vi "FPGA IO.vi"() -> ()   [LabVIEW 2012]
doc: "Accepts inputs from a host based VI for controlling analog and digital outputs on a R-series board containing an FPGA. This VI will produce 4 different signal types dependent on the user input and the channel of interest. When the <B>WaveType</B> is set to laser, the first three channels will produce either a sine or square wave at the frequency <B>f0</B> while the last two produce only square waves. When the wavetype is set to speaker or none, all channels produce the same signal (although for the speaker, signals with a gain of <B>Amp</B> applied)."
uses:
  <vilib>/Platform/TimedLoop/XDataNode/XDataNode.xnode
  <vilib>/Platform/TimedLoop/XDataNode/nitl_modes.ctl
  <vilib>/Platform/TimedLoop/XDataNode/XDNodeRunTimeDep.lvlib
  <vilib>/Platform/TimedLoop/XDataNode/wakeup.ctl
  <vilib>/Platform/TimedLoop/XDataNode/timing_clust.ctl
  <vilib>/eio/EIONode/EIONode.xnode
  <vilib>/rvi/FXPMathLib/FxpMul/XNode/nifxpmath_Multiplier.xnode
  <vilib>/rvi/FXPMathLib/FxpAdd/XNode/nifxpmath_Add.xnode
  <vilib>/rvi/eio/common/nirviEmuTemplateMethod_errors.vi
  <vilib>/rvi/FXPMathLib/sim/FxpSim.dll
  Controls/FxdPt Props.ctl
  Controls/FPGA Signal.ctl
  Reusable/PAS/Main/Controls/Laser Modulation.ctl
panel:
  in  "LaserEn":T1
  in  "Laser Switch":bool
  out "OtherOut":T2
  in  "Cell 5":T3
  in  "Cell 4":T3
  in  "Cell 3":T3
  in  "Cell 2":T3
  in  "Cell 1":T3
  in  "wType":T5
  out "Stopped":bool
  out "SquareOut":T2
  in  "stop":bool
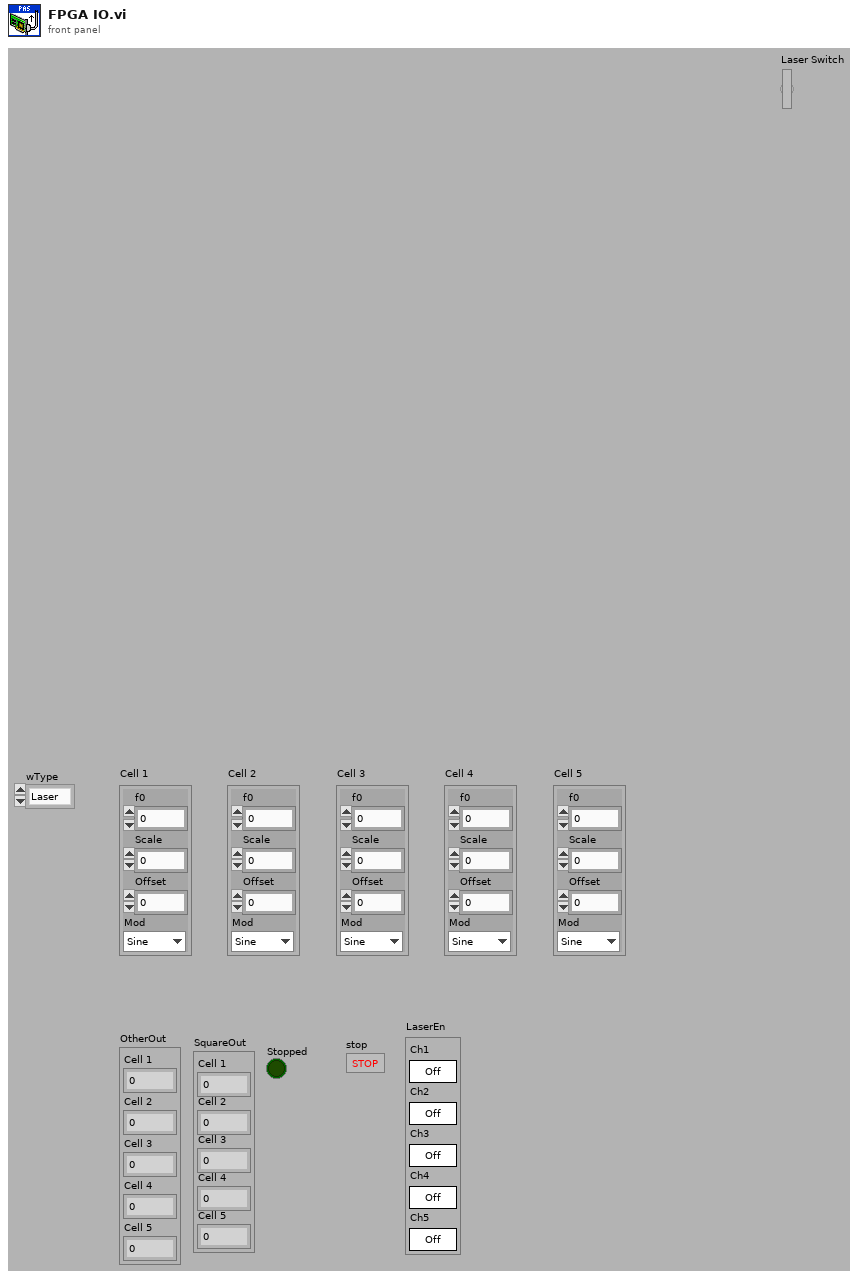
[diagram p1: front panel]
types:
  T1 = cluster{"Ch1":bool, "Ch2":bool, "Ch3":bool, "Ch4":bool, "Ch5":bool}
  T2 = cluster{"Cell 1":i16, "Cell 2":i16, "Cell 3":i16, "Cell 4":i16, "Cell 5":i16}
  T3 = typedef "FxdPt Props.ctl" = cluster{"f0":fxp<+,32,0>, "Scale":fxp<+,14,1>, "Offset":i16, "Mod":T4}
  T4 = typedef "Laser Modulation.ctl" = enum8{"Sine", "Square"}
  T5 = typedef "FPGA Signal.ctl" = enum16{"Laser", "None", "Speaker"}
  T6 = typedef "XDNodeRunTimeDep.lvlib/timing_clust.ctl" = cluster{"Expected End [f-1]":u64, "Actual End [f-1]":u64, "Finished Late? [f-1]":bool, "Expected End [i-1]":u64, "Actual End [i-1]":u64, "Finished Late? [i-1]":bool, "Expected Start [i]":u64, "Actual Start [i]":u64, "Expected Start [f]":u64, "Actual Start [f]":u64, "Source Name":string, "Structure Name":string, "Period":i64, "Deadline":i64, "Offset":i64, "Start":i64, "Priority":i32, "Timeout":i32, "Mode":T7, "Wakeup Reason":T8, "Error":errorcluster, "Source Type":string, "Secondary Source Type":string, "Global End Time":u64, "Global Start Time":u64, "Frame Duration":u64, "Iteration Duration":u64, "Assigned CPU":i32, "I/O Scan Engine Mode":u32}
  T7 = typedef "XDNodeRunTimeDep.lvlib/nitl_modes.ctl" = enum32{"No Change", "Process missed periods, maintain original phase", "Discard missed periods, maintain original phase", "Process missed periods, ignore original phase", "Discard missed periods, ignore original phase"}
  T8 = typedef "XDNodeRunTimeDep.lvlib/wakeup.ctl" = enum32{"Normal", "Aborted", "Asynchronous wakeup", "Timing source error", "Timed loop error", "Timeout"}
  T9 = cluster{"square wave out":i16, "square wave out":i16, "square wave out":i16, "square wave out":i16, "square wave out":i16}
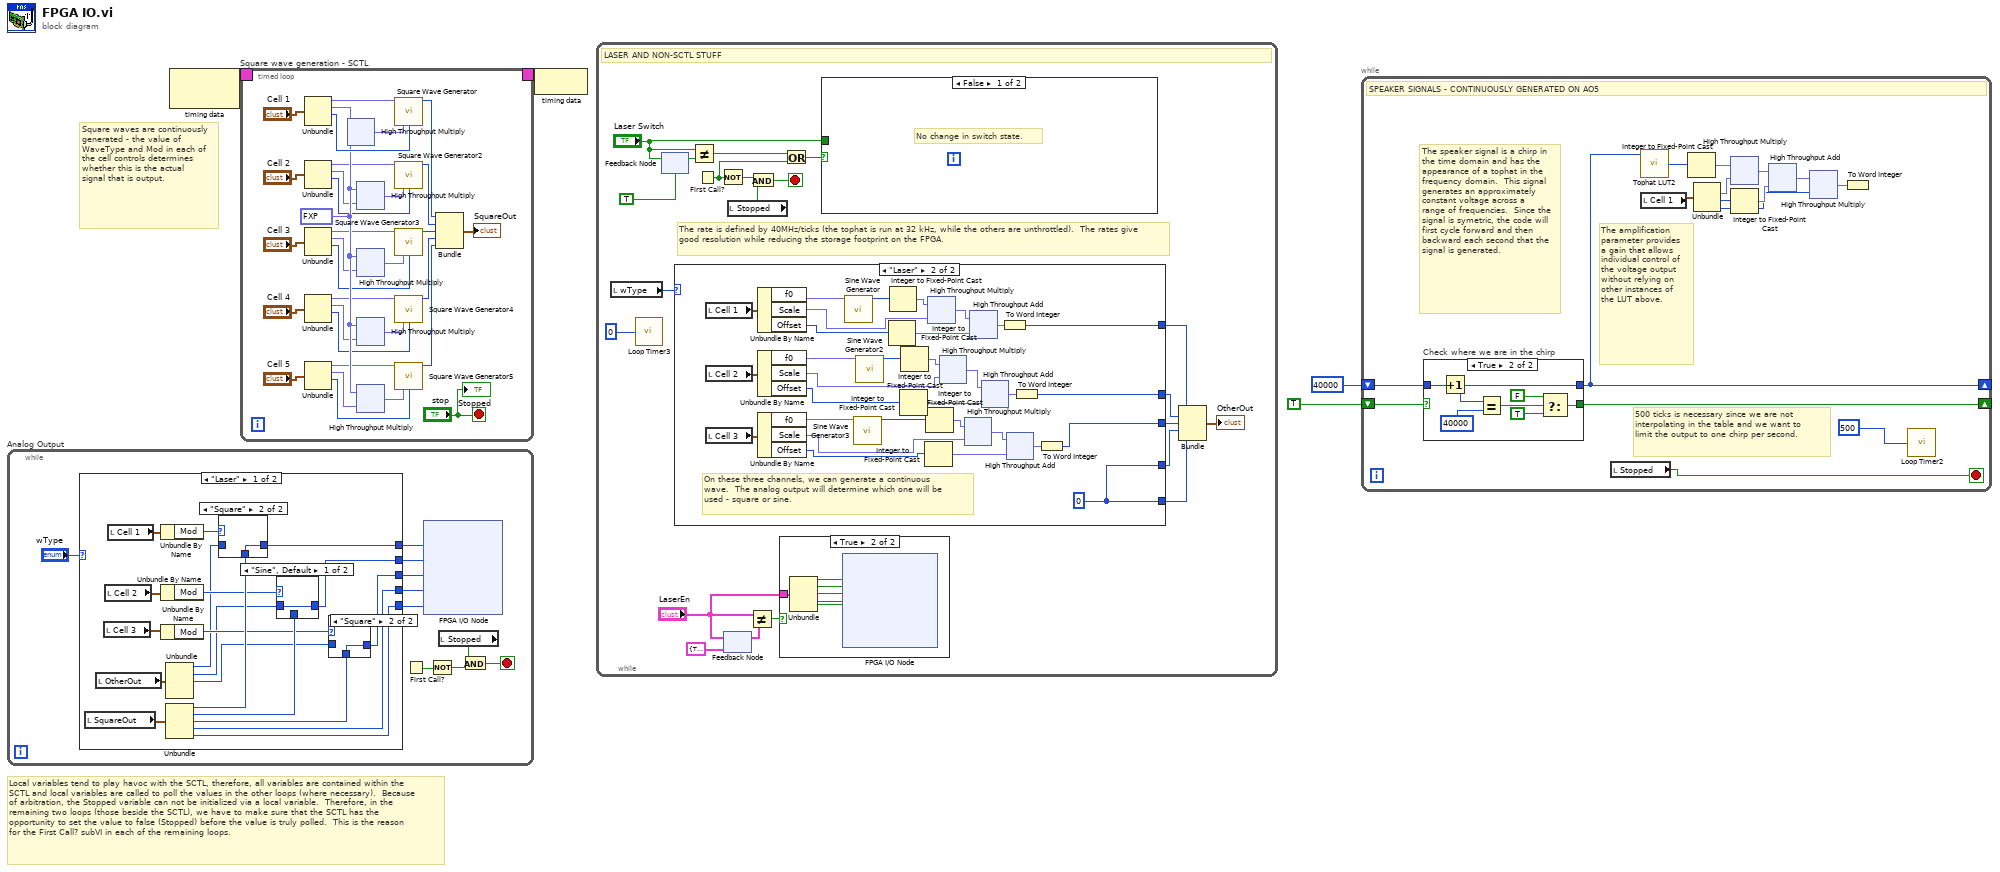
[diagram p0: block diagram]
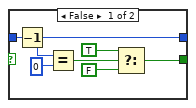
[diagram p2: hidden frame]
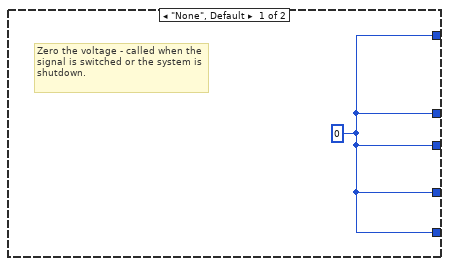
[diagram p4: hidden frame]
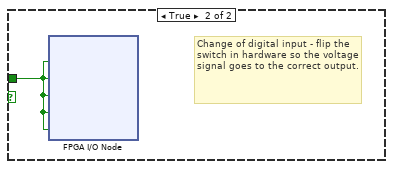
[diagram p5: hidden frame]
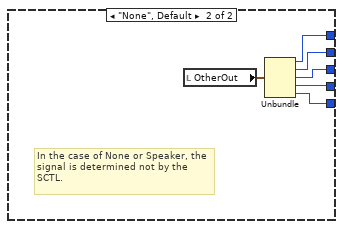
[diagram p9: hidden frame]
diagram:
  # "Square waves are continuously generated - the value of WaveType and Mod in each of the cell controls determines whether this is the actual signal that is output."
  # "Local variables tend to play havoc with the SCTL, therefore, all variables are contained within the SCTL and local variables are called to poll the values in the other loops (where necessary).  Because of arbitration, the Stopped variable can not be initialized via a local variable.  Therefore, in the remaining two loops (those beside the SCTL), we have to make sure that the SCTL has the opportunity to set the value to false (Stopped) before the value is truly polled.  This is the reason for the First Call? subVI in each of the remaining loops."
  n1 = while "Analog Output" {
    stop <- w5 stop-if-true
    n2 = case shown="\"Laser\"" "wType" {
      tunnel: [w26 w44] -> w14
      tunnel: [w16 w43] -> w13
      tunnel: [w15 w42] -> w12
      tunnel: [w31 w41] -> w11
      tunnel: [w32 w40] -> w10
      frame "Laser" {
        n3 = local read "SquareOut"() -> (w33:T2)
        n4 = local read "OtherOut"() -> (w30:T2)
        n5 = local read "Cell 3"() -> (w22:T3)
        n6 = local read "Cell 2"() -> (w24:T3)
        n7 = local read "Cell 1"() -> (w29:T3)
        n8 = Unbundle By Name(w29) -> ("Mod"=w28:T4)
        n9 = Unbundle By Name(w24) -> ("Mod"=w23:T4)
        n10 = Unbundle By Name(w22) -> ("Mod"=w21:T4)
        n11 = Unbundle(w30) -> ("Cell 1"=w17:i16, "Cell 2"=w18:i16, "Cell 3"=w19:i16)  [unwired: 2 out]
        n12 = Unbundle(w33) -> ("Cell 1"=w27:i16, "Cell 2"=w25:i16, "Cell 3"=w20:i16, "Cell 4"=w31:i16, "Cell 5"=w32:i16)
        n13 = case shown="\"Square\"" w28 {
          tunnel: w27 -> [_ w39]
          tunnel: [w38 w39] -> w26
          tunnel: w17 -> [w38 _]
          frame "Sine", Default {
          }
          frame "Square" {
          }
        }
        n14 = case shown="\"Sine\", Default" w23 {
          tunnel: w25 -> [_ w37]
          tunnel: [w36 w37] -> w16
          tunnel: w18 -> [w36 _]
          frame "Sine", Default {
          }
          frame "Square" {
          }
        }
        n15 = case shown="\"Square\"" w21 {
          tunnel: w20 -> [_ w35]
          tunnel: [w34 w35] -> w15
          tunnel: w19 -> [w34 _]
          frame "Sine", Default {
          }
          frame "Square" {
          }
        }
      }
      frame "None", Default {
        # "In the case of None or Speaker, the signal is determined not by the SCTL."
        n16 = local read "OtherOut"() -> (w45:T2)
        n17 = Unbundle(w45) -> ("Cell 1"=w44:i16, "Cell 2"=w43:i16, "Cell 3"=w42:i16, "Cell 4"=w41:i16, "Cell 5"=w40:i16)
      }
    }
    n18 = First Call?() -> (First Call?: T/F=w8:bool)
    n19 = xnode "FPGA I/O Node"("Ch 1 AO"=w14, "Ch 2 AO"=w13, "Ch 3 AO"=w12, "Ch 4 AO"=w11, "Ch 5 AO"=w10) -> ()  [unwired: 5 in, 5 out]
    n20 = Not(x=w8) -> (.not. x?=w6:bool)
    n21 = local read "Stopped"() -> (w7:bool)
    n22 = And(x=w7, y=w6) -> (x .and. y?=w5:bool)
  }
  n23 = node-c288() -> (w4:T6)  [unwired: 1 in]
  n24 = timed-loop "Square wave generation - SCTL" {
    timing: w4 -> [_]
    timing-out: [_] -> w3
    stop <- "stop" stop-if-true
    w66 = fxp<+,15,15> 32767.0 ("n")
    n25 = Unbundle("Cell 1") -> ("f0"=w69:fxp<+,32,0>, "Scale"=w68:fxp<+,14,1>, "Offset"=w67:i16)  [unwired: 1 out]
    n26 = Unbundle("Cell 2") -> ("f0"=w57:fxp<+,32,0>, "Scale"=w56:fxp<+,14,1>, "Offset"=w58:i16)  [unwired: 1 out]
    n27 = Unbundle("Cell 3") -> ("f0"=w54:fxp<+,32,0>, "Scale"=w55:fxp<+,14,1>, "Offset"=w59:i16)  [unwired: 1 out]
    n28 = Unbundle("Cell 4") -> ("f0"=w53:fxp<+,32,0>, "Scale"=w52:fxp<+,14,1>, "Offset"=w60:i16)  [unwired: 1 out]
    n29 = Unbundle("Cell 5") -> ("f0"=w47:fxp<+,32,0>, "Scale"=w46:fxp<+,14,1>, "Offset"=w61:i16)  [unwired: 1 out]
    n30 = xnode "High Throughput Multiply"("x"=w68, "y"=w66) -> ("x*y"=w71:fxp<+,29,16>)
    n31 = xnode "High Throughput Multiply"("x"=w66, "y"=w56) -> ("x*y"=w49:fxp<+,29,16>)
    n32 = xnode "High Throughput Multiply"("x"=w66, "y"=w55) -> ("x*y"=w50:fxp<+,29,16>)
    n33 = xnode "High Throughput Multiply"("x"=w66, "y"=w52) -> ("x*y"=w51:fxp<+,29,16>)
    n34 = xnode "High Throughput Multiply"("x"=w66, "y"=w46) -> ("x*y"=w48:fxp<+,29,16>)
    n35 = call "Square Wave Generator"("frequency (periods/tick)"=w69, "amplitude"=w71, "offset"=w67) -> ("square wave out"=w78:i16)  [unwired: 12 in]
    n36 = call "Square Wave Generator2"("frequency (periods/tick)"=w57, "amplitude"=w49, "offset"=w58) -> ("square wave out"=w77:i16)  [unwired: 12 in]
    n37 = call "Square Wave Generator3"("frequency (periods/tick)"=w54, "amplitude"=w50, "offset"=w59) -> ("square wave out"=w76:i16)  [unwired: 12 in]
    n38 = call "Square Wave Generator4"("frequency (periods/tick)"=w53, "amplitude"=w51, "offset"=w60) -> ("square wave out"=w75:i16)  [unwired: 12 in]
    n39 = call "Square Wave Generator5"("frequency (periods/tick)"=w47, "amplitude"=w48, "offset"=w61) -> ("square wave out"=w74:i16)  [unwired: 12 in]
    n40 = Bundle("square wave out"=w78, "square wave out"=w77, "square wave out"=w76, "square wave out"=w75, "square wave out"=w74) -> (→"SquareOut":T9)  [unwired: 1 in]
    "Stopped" <- "stop"
  }
  n41 = node-c288(w3) -> ()
  n42 = while {
    stop <- w101 stop-if-true
    # "The rate is defined by 40MHz/ticks (the tophat is run at 32 kHz, while the others are unthrottled).  The rates give good resolution while reducing the storage footprint on the FPGA."
    # "LASER AND NON-SCTL STUFF"
    n43 = local read "wType"() -> (w93:T5)
    n44 = call "Loop Timer3"("Count(Ticks)"=u32 0) -> ()  [unwired: 1 out]
    n45 = feedback-in #1("Laser Switch") -> ()
    n46 = feedback #1(TRUE ("Drive")) -> (w98:bool)
    n47 = case shown="\"Laser\"" w93 {
      tunnel: [w108 w109] -> w96
      tunnel: [w108 w110] -> w97
      tunnel: [w108 w111] -> w95
      tunnel: [w108 w139] -> w87
      tunnel: [w108 w139] -> w86
      frame "None", Default {
        w108 = i16 0
        # "Zero the voltage - called when the signal is switched or the system is shutdown."
      }
      frame "Laser" {
        w139 = i16 0
        # "On these three channels, we can generate a continuous wave.  The analog output will determine which one will be used - square or sine."
        n48 = local read "Cell 1"() -> (w133:T3)
        n49 = local read "Cell 2"() -> (w124:T3)
        n50 = local read "Cell 3"() -> (w112:T3)
        n51 = Unbundle By Name(w133) -> ("f0"=w132:fxp<+,32,0>, "Scale"=w131:fxp<+,14,1>, "Offset"=w130:i16)
        n52 = Unbundle By Name(w124) -> ("f0"=w123:fxp<+,32,0>, "Scale"=w122:fxp<+,14,1>, "Offset"=w121:i16)
        n53 = Unbundle By Name(w112) -> ("f0"=w118:fxp<+,32,0>, "Scale"=w119:fxp<+,14,1>, "Offset"=w120:i16)
        n54 = call "Sine Wave Generator"("frequency (periods/tick)"=w132) -> ("sine out"=w136:i16)  [unwired: 14 in]
        n55 = call "Sine Wave Generator3"("frequency (periods/tick)"=w118) -> ("sine out"=w115:i16)  [unwired: 14 in]
        n56 = call "Sine Wave Generator2"("frequency (periods/tick)"=w123) -> ("sine out"=w127:i16)  [unwired: 14 in]
        n57 = Integer to Fixed-Point Cast(integer=w130) -> (fixed-point=w134:fxp<+/-,16,16>)  [unwired: 1 in]
        n58 = Integer to Fixed-Point Cast(integer=w136) -> (fixed-point=w135:fxp<+/-,16,16>)  [unwired: 1 in]
        n59 = Integer to Fixed-Point Cast(integer=w121) -> (fixed-point=w129:fxp<+/-,16,16>)  [unwired: 1 in]
        n60 = Integer to Fixed-Point Cast(integer=w127) -> (fixed-point=w128:fxp<+/-,16,16>)  [unwired: 1 in]
        n61 = Integer to Fixed-Point Cast(integer=w120) -> (fixed-point=w113:fxp<+/-,16,16>)  [unwired: 1 in]
        n62 = Integer to Fixed-Point Cast(integer=w115) -> (fixed-point=w114:fxp<+/-,16,16>)  [unwired: 1 in]
        n63 = xnode "High Throughput Multiply"("x"=w135, "y"=w131) -> ("x*y"=w138:fxp<+/-,30,17>)
        n64 = xnode "High Throughput Multiply"("x"=w128, "y"=w122) -> ("x*y"=w125:fxp<+/-,30,17>)
        n65 = xnode "High Throughput Multiply"("x"=w114, "y"=w119) -> ("x*y"=w117:fxp<+/-,30,17>)
        n66 = xnode "High Throughput Add"("x"=w138, "y"=w134) -> ("x+y"=w137:fxp<+/-,16,16>)
        n67 = xnode "High Throughput Add"("x"=w125, "y"=w129) -> ("x+y"=w126:fxp<+/-,16,16>)
        n68 = To Word Integer(number=w137) -> (16bit integer=w109:i16)
        n69 = xnode "High Throughput Add"("x"=w117, "y"=w113) -> ("x+y"=w116:fxp<+/-,16,16>)
        n70 = To Word Integer(number=w126) -> (16bit integer=w110:i16)
        n71 = To Word Integer(number=w116) -> (16bit integer=w111:i16)
      }
    }
    n72 = Not Equal?(x="Laser Switch", y=w98) -> (x != y?=w92:bool)
    n73 = First Call?() -> (First Call?: T/F=w90:bool)
    n74 = Not(x=w90) -> (.not. x?=w89:bool)
    n75 = feedback-in #2("LaserEn") -> ()
    n76 = feedback #2(T1 {"Ch1"=TRUE, "Ch2"=TRUE, "Ch3"=TRUE, "Ch4"=TRUE, "Ch5"=TRUE} ("LaserEn")) -> (w85:T1)
    n77 = local read "Stopped"() -> (w91:bool)
    n78 = Not Equal?(x="LaserEn", y=w85) -> (x != y?=w83:bool)
    n79 = And(x=w89, y=w91) -> (x .and. y?=w101:bool)
    n80 = case shown="True" w83 {
      tunnel: "LaserEn" -> [_ w107]
      frame False {
      }
      frame True {
        n81 = Unbundle(w107) -> ("Ch1"=w106:bool, "Ch2"=w105:bool, "Ch3"=w104:bool, "Ch4"=w103:bool, "Ch5"=w102:bool)
        n82 = xnode "FPGA I/O Node"("Ch 1 Enable"=w106, "Ch 2 Enable"=w105, "Ch 3 Enable"=w104, "Ch 4 Enable"=w103, "Ch 5 Enable"=w102) -> ()  [unwired: 5 in, 5 out]
      }
    }
    n83 = Or(x=w92, y=w90) -> (x .or. y?=w100:bool)
    n84 = case shown="False" w100 {
      tunnel: "Laser Switch" -> [_ w140]
      frame False {
        # "No change in switch state."
      }
      frame True {
        # "Change of digital input - flip the switch in hardware so the voltage signal goes to the correct output."
        n85 = xnode "FPGA I/O Node"("Spk Sel 2"=w140, "Spk Sel 1"=w140, "Spk Sel 3"=w140, "Spk Sel 4"=w140, "Spk Sel 5"=w140) -> ()  [unwired: 5 in, 5 out]
      }
    }
    n86 = Bundle(w96, w97, w95, w86, w87) -> (→"OtherOut":cluster{i16, i16, i16, i16, i16})  [unwired: 1 in]
  }
  n87 = while {
    shift-right: [w155] -> _
    shift-left: u32 40000 -> [w156]
    shift-right: [w143] -> _
    shift-left: TRUE -> [w144]
    stop <- w141 stop-if-true
    # "500 ticks is necessary since we are not interpolating in the table and we want to limit the output to one chirp per second."
    # "The amplification parameter provides a gain that allows individual control of the voltage output without relying on other instances of the LUT above."
    # "The speaker signal is a chirp in the time domain and has the appearance of a tophat in the frequency domain.  This signal generates an approximately constant voltage across a range of frequencies.  Since the signal is symetric, the code will first cycle forward and then backward each second that the signal is generated."
    # "SPEAKER SIGNALS - CONTINUOUSLY GENERATED ON AO5"
    n88 = case "Check where we are in the chirp" shown="True" w144 {
      tunnel: w156 -> [w159 w170]
      tunnel: [w158 w165] -> w143
      tunnel: [w157 w164] -> w155
      frame False {
        n89 = Decrement(x=w159) -> (x-1=w157:u32)
        n90 = Equal?(x=w157, y=u32 0) -> (x = y?=w161:bool)
        n91 = Select(t=TRUE, s=w161, f=FALSE) -> (s? t:f=w158:bool)
      }
      frame True {
        n92 = Increment(x=w170) -> (x+1=w164:u32)
        n93 = Equal?(x=w164, y=u32 40000) -> (x = y?=w168:bool)
        n94 = Select(t=FALSE, s=w168, f=TRUE) -> (s? t:f=w165:bool)
      }
    }
    n95 = local read "Stopped"() -> (w141:bool)
    n96 = call "Tophat LUT2"("address"=w155) -> ("data out"=w151:i16)  [unwired: 1 in, 7 out]
    n97 = local read "Cell 1"() -> (w145:T3)
    n98 = Integer to Fixed-Point Cast(integer=w151) -> (fixed-point=w150:fxp<+/-,16,16>)  [unwired: 1 in]
    n99 = Unbundle(w145) -> ("Scale"=w149:fxp<+,14,1>, "Offset"=w153:i16, "Mod"=w146:T4)  [unwired: 1 out]
    n100 = xnode "High Throughput Multiply"("x"=w150, "y"=w149) -> ("x*y"=w154:fxp<+/-,30,17>)
    n101 = Integer to Fixed-Point Cast(integer=w153) -> (fixed-point=w152:fxp<+/-,16,16>)  [unwired: 1 in]
    n102 = xnode "High Throughput Add"("x"=w154, "y"=w152) -> ("x+y"=w148:fxp<+/-,31,18>)
    n103 = xnode "High Throughput Multiply"("x"=w148, "y"=w146) -> ("x*y"=w147:fxp<+/-,16,16>)
    n104 = To Word Integer(number=w147) -> ()  [unwired: 1 out]
    n105 = call "Loop Timer2"("Count(Ticks)"=u32 500) -> ()  [unwired: 1 out]
  }
